vi "Load Save Frequency Correction Table.vi"(0 "VISA resource name":refnum<visa-resource-name>, 5 "Correction Table Operation (0:Save)":i32(ring) items=["Save", "Recall"], 9 "Filename (Test)":string="Test", 11 "error in (no error)":errorcluster, 12 "Drive (D)":string="D") -> (4 "VISA resource name out":refnum<visa-resource-name>, 15 "error out":errorcluster)   [LabVIEW 2020, in "Anritsu Signal Analyzer Series.lvlib"]
doc: "Loads or Saves the level frequency correction table of the spectrum analyzer."
uses:
  Anritsu Signal Analyzer Series.lvlib
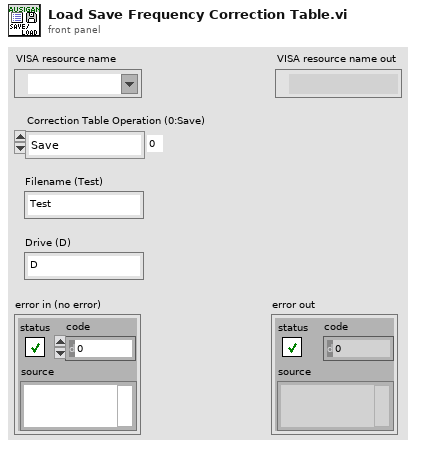
[diagram p1: front panel]
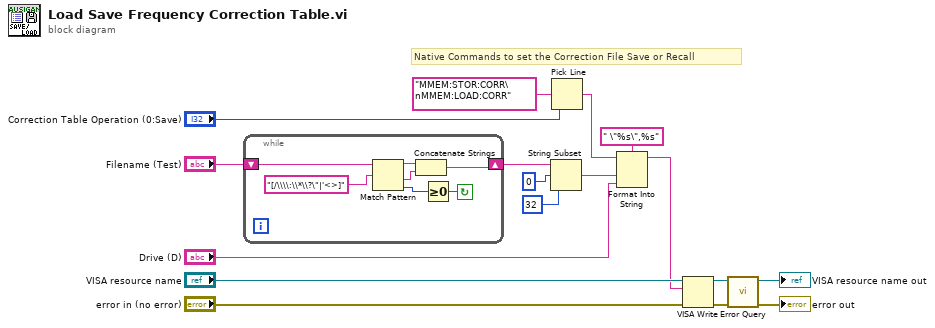
[diagram p0: block diagram]
diagram:
  # "Native Commands to set the Correction File Save or Recall"
  n1 = while {
    shift-right: [w20] -> w10
    shift-left: "Filename (Test)" -> [w19]
    stop <- w23 continue-if-true
    n2 = Match Pattern(string=w19, regular expression="[/\\\\:\\*\\?\"|'<>]") -> (before substring=w22:string, after substring=w21:string, offset past match=w24:i32)  [unwired: 1 in, 1 out]
    n3 = Concatenate Strings(w22, w21) -> (w20:string)
    n4 = Greater Or Equal To 0?(x=w24) -> (x >= 0?=w23:bool)
  }
  n5 = String Subset(string=w10, offset (0)=0, length (rest)=32 ("length (rest)")) -> (substring=w11:string)
  n6 = Pick Line(multi-line string="MMEM:STOR:CORR\nMMEM:LOAD:CORR" ("_Command"), line index="Correction Table Operation (0:Save)") -> (output string=w3:string)  [unwired: 1 in]
  n7 = Format Into String(format string=" \"%s\",%s", initial string=w3, w11, "Drive (D)") -> (resulting string=w1:string)  [unwired: 1 in, 1 out]
  n8 = VISA Write(VISA resource name="VISA resource name", write buffer=w1, error in (no error)="error in (no error)") -> (VISA resource name out=w6:refnum<visa-resource-name>, error out=w5:errorcluster)  [unwired: 1 out]
  n9 = call "Error Query.vi"("error in (no error)"=w5, "VISA resource name"=w6) -> ("error out"=→"error out":errorcluster, "VISA resource name out"=→"VISA resource name out":refnum<visa-resource-name>)  [unwired: 6 in, 2 out]
